vi "MainOLD.vi"() -> ()   [LabVIEW 2016]
uses:
  MainFGV/MainFGV_mods.ctl
  Log/log_mods.ctl
panel:
  in  "advancedConfig":bool
  in  "Start":bool
  in  "clear":bool
  in  "simulation":bool
  in  "Log":string
  in  "tab":enum32{"Sinal no tempo", "Espectro"}(tab)
  out "contData":dbl[][](graph) caption="Continuo"
  out "levels":cluster{"Array":i32[], "Array":dbl[]}(graph) caption="XY Graph"
  out "timeData":dbl[][](graph) caption="RMS"
  out "spec":waveform(dbl)[](graph) caption="Espectro"
  in  "stop":bool
  in  "TestName":string caption="Nome do ensaio"
  in  "config":bool
  in  "TesrtDir":path=path "C:/Users/admin/Desktop/Teste" caption="Diretório do ensaio"
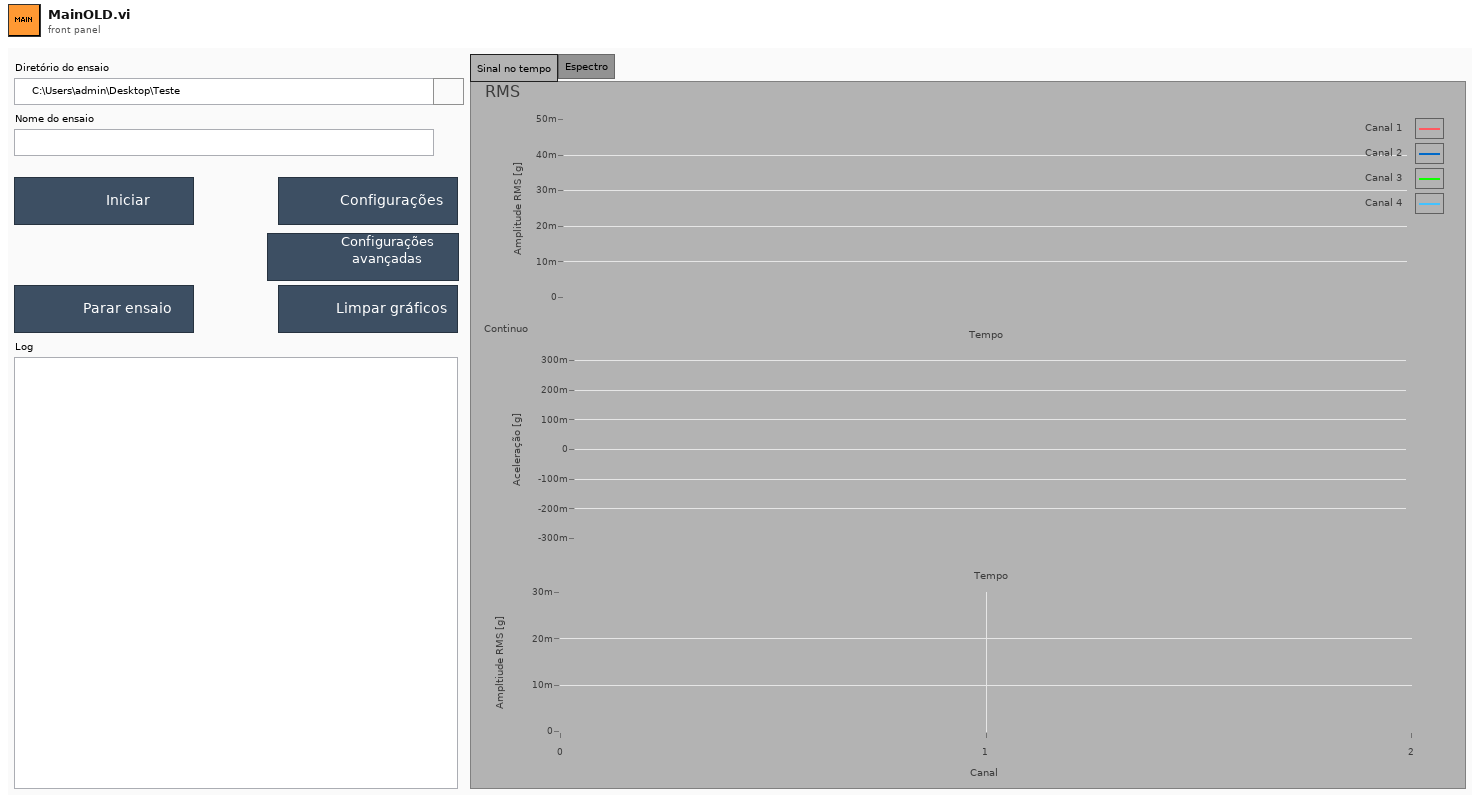
[diagram p1: front panel]
types:
  T1 = typedef "log_mods.ctl" = enum16{"Init", "LogFileRefnum", "SetStatus", "WriteAcel", "WriteToLog", "End"}
  T2 = typedef "MainFGV_mods.ctl" = enum16{"Init", "Config", "Advanced", "CreateTask", "Register", "Acquire", "Start", "Burst", "Record", "End"}
  T3 = cluster{"simulation":bool, "TesrtDir":path, "TestName":string}
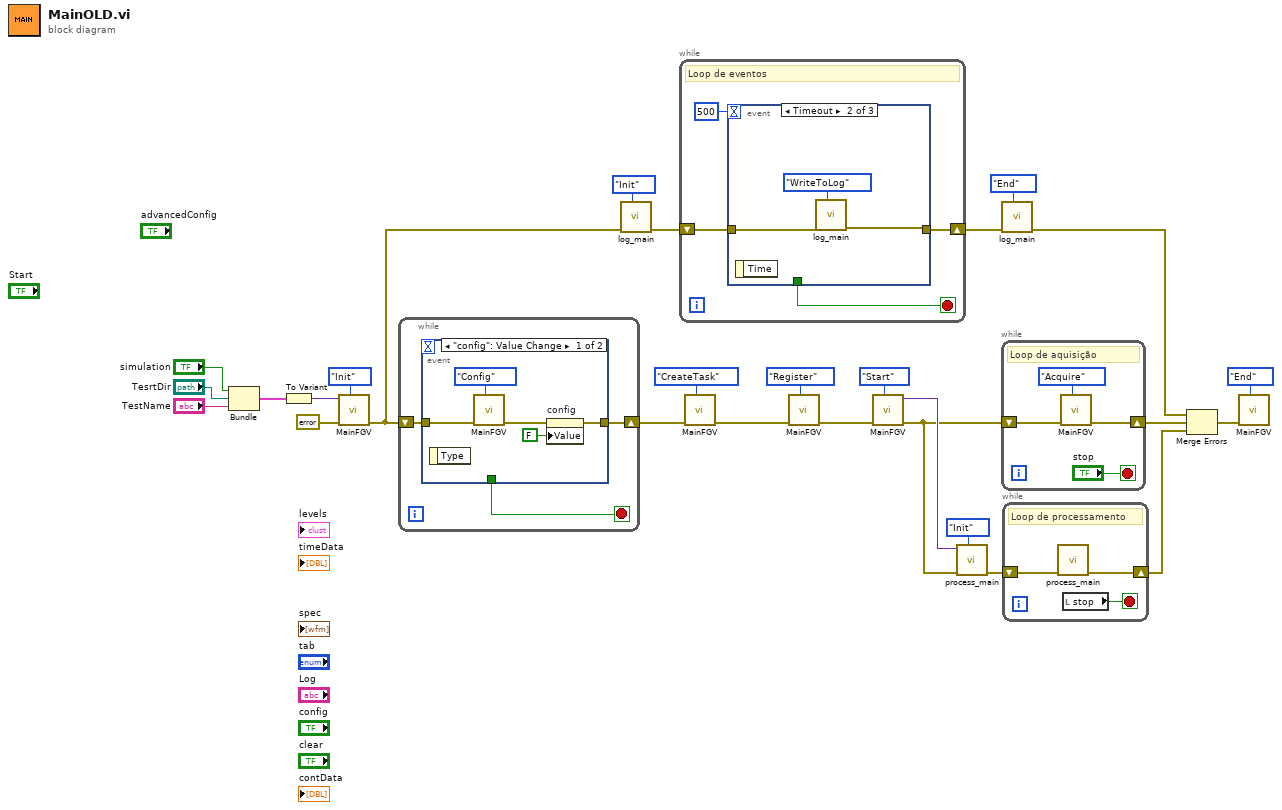
[diagram p0: block diagram]
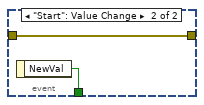
[diagram p2: hidden frame]
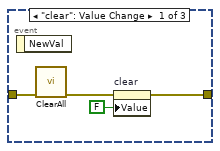
[diagram p3: hidden frame]
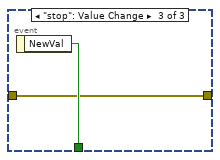
[diagram p4: hidden frame]
diagram:
  n1 = Bundle("simulation"="simulation", "TesrtDir"="TesrtDir", "TestName"="TestName") -> (w24:T3)  [unwired: 1 in]
  n2 = To Variant(anything=w24) -> (Variant=w23:variant)
  n3 = call "MainFGV.vi"("FGV_mods"=MainFGV_mods."Init", "Error In"=errorcluster {"status"=FALSE, "code"=0, "source"=""}, "DataIn"=w23) -> ("Error Out"=w7:errorcluster)  [unwired: 7 in, 1 out]
  n4 = while {
    shift-right: [w29] -> w19
    shift-left: w7 -> [w30]
    stop <- w28 stop-if-true
    n5 = event shown="[0] \"config\": Value Change" {
      selector: _ -> [_ _]
      dyn-events: _ -> [_ _]
      timeout: _ -> [_ _]
      tunnel: w30 -> [w34 w36]
      tunnel: [w32 w36] -> w29
      tunnel: [_ w37] -> w28
      event "config": Value Change {
        n6 = event-data() -> ()  [unwired: 1 in, 1 out]
        n7 = call "MainFGV.vi"("FGV_mods"=MainFGV_mods."Config", "Error In"=w34) -> ("Error Out"=w33:errorcluster)  [unwired: 8 in, 1 out]
        n8 = property on="config" class="Bool (strict)"(error in=w33, "Value"=FALSE ("config")) -> (error out=w32:errorcluster)  [unwired: 1 in, 1 out]
      }
      event "Start": Value Change {
        n9 = event-data() -> ("NewVal"=w37:bool)  [unwired: 1 in]
      }
    }
  }
  n10 = call "log_main.vi"("FGV_mods"=log_mods."Init", "Error In"=w7) -> ("Error Out"=w1:errorcluster)  [unwired: 8 in, 1 out]
  n11 = while {
    shift-right: [w40] -> w3
    shift-left: w1 -> [w41]
    stop <- w39 stop-if-true
    # "Loop de eventos"
    n12 = event shown="[1] Timeout" {
      selector: _ -> [_ _ _]
      dyn-events: _ -> [_ _ _]
      timeout: 500 -> [_ _ _]
      tunnel: w41 -> [w45 w47 w49]
      tunnel: [w43 w46 w49] -> w40
      tunnel: [_ _ w50] -> w39
      event "clear": Value Change {
        n13 = event-data() -> ()  [unwired: 1 in, 1 out]
        n14 = call "ClearAll.vi"("error in"=w45) -> ("error out"=w44:errorcluster)  [unwired: 10 in]
        n15 = property on="clear" class="Bool (strict)"(error in=w44, "Value"=FALSE ("clear")) -> (error out=w43:errorcluster)  [unwired: 1 in, 1 out]
      }
      event Timeout {
        n16 = event-data() -> ()  [unwired: 1 in, 1 out]
        n17 = call "log_main.vi"("FGV_mods"=log_mods."WriteToLog", "Error In"=w47) -> ("Error Out"=w46:errorcluster)  [unwired: 8 in, 1 out]
      }
      event "stop": Value Change {
        n18 = event-data() -> ("NewVal"=w50:bool)  [unwired: 1 in]
      }
    }
  }
  n19 = call "MainFGV.vi"("FGV_mods"=MainFGV_mods."CreateTask", "Error In"=w19) -> ("Error Out"=w17:errorcluster)  [unwired: 8 in, 1 out]
  n20 = call "MainFGV.vi"("FGV_mods"=MainFGV_mods."Register", "Error In"=w17) -> ("Error Out"=w15:errorcluster)  [unwired: 8 in, 1 out]
  n21 = call "MainFGV.vi"("FGV_mods"=MainFGV_mods."Start", "Error In"=w15) -> ("Error Out"=w5:errorcluster, "DataOut"=w9:variant)  [unwired: 8 in]
  n22 = call "process_main.vi"("FGV_mods"=enum16{"Init", "Exec", "End"}."Init", "Error In"=w5, "DataIn"=w9) -> ("Error Out"=w8:errorcluster)  [unwired: 7 in, 1 out]
  n23 = call "log_main.vi"("FGV_mods"=log_mods."End", "Error In"=w3) -> ("Error Out"=w2:errorcluster)  [unwired: 8 in, 1 out]
  n24 = while {
    shift-right: [w51] -> w13
    shift-left: w5 -> [w52]
    stop <- "stop" stop-if-true
    # "Loop de aquisição"
    n25 = call "MainFGV.vi"("FGV_mods"=MainFGV_mods."Acquire", "Error In"=w52) -> ("Error Out"=w51:errorcluster)  [unwired: 8 in, 1 out]
  }
  n26 = while {
    shift-right: [w55] -> w12
    shift-left: w8 -> [w56]
    stop <- w57 stop-if-true
    # "Loop de processamento"
    n27 = call "process_main.vi"("Error In"=w56) -> ("Error Out"=w55:errorcluster)  [unwired: 9 in, 1 out]
    n28 = local read "stop"() -> (w57:bool)
  }
  n29 = Merge Errors(w2, w13, w12) -> (w11:errorcluster)
  n30 = call "MainFGV.vi"("FGV_mods"=MainFGV_mods."End", "Error In"=w11) -> ()  [unwired: 8 in, 2 out]
